vi "探头数据读取.vi"(11 "编号":string) -> ()   [LabVIEW 2016, in "斯坦道多参数.lvlib"]
panel:
  out "日期/时间字符串 2":string
  out "日期/时间字符串":string
  out "运行状态":u16(ring) items=["空闲", "水样测试", "标样核查"]
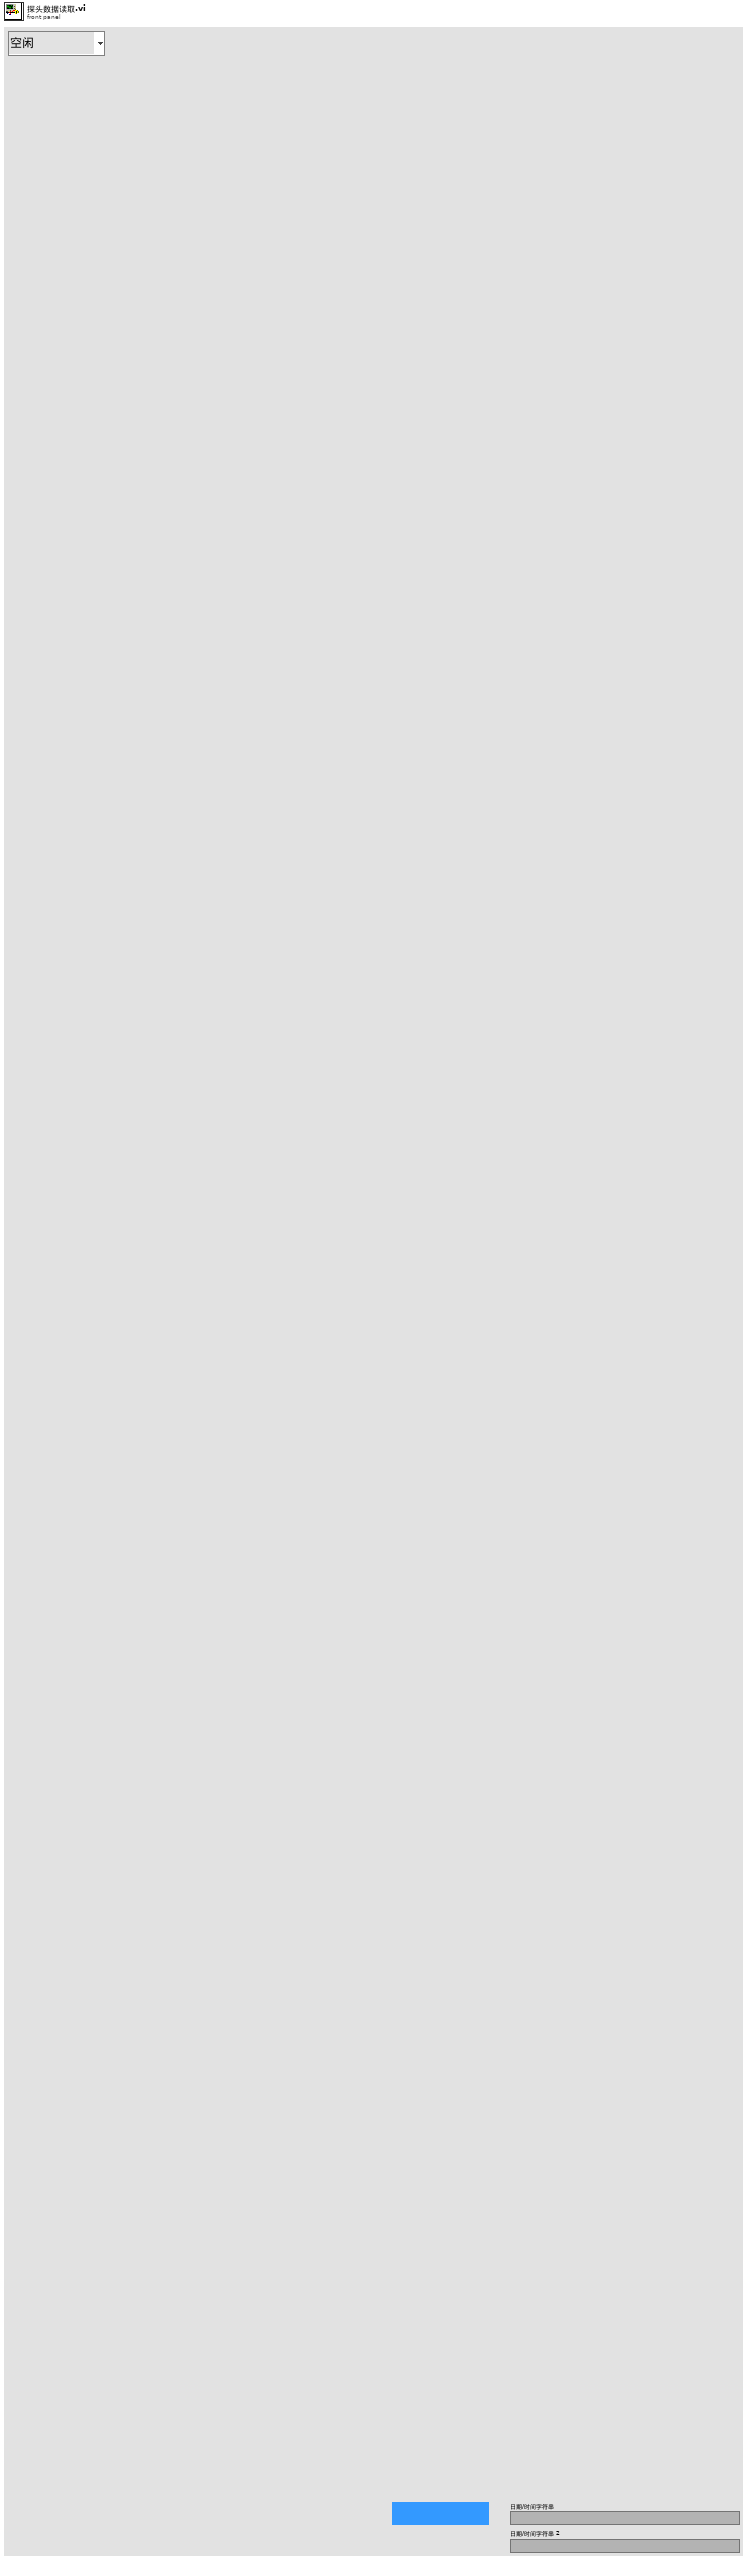
[diagram p1: front panel]
types:
  T1 = typedef "斯坦道多参数.lvlib/通知队列类型.ctl" = enum16{"pH", "DO", "DO2", "Cond", "Turb", "ORP", "叶绿素a", "藻密度", "COD", "氯化物", "氨氮", "水中油"}
  T2 = cluster{"温度测量值":sgl, "测量值":sgl, "温度偏移修正值":sgl, "信号值":sgl, "数据标识":string}
  T3 = cluster{"温度测量值":sgl, "DO%":sgl, "DOmg/L":sgl, "温度偏移修正值":sgl, "数据标识mg/L":string, "数据标识%":string}
  T4 = cluster{"水温 (℃)":cluster{"量程下限":dbl, "量程上限":dbl}, "DO (mg/L)":cluster{"量程下限":dbl, "量程上限":dbl}, "DO (%)":cluster{"量程下限":dbl, "量程上限":dbl}, "pH":cluster{"量程下限":dbl, "量程上限":dbl}, "电导率 (μS/cm)":cluster{"量程下限":dbl, "量程上限":dbl}, "盐度":cluster{"量程下限":dbl, "量程上限":dbl}, "浊度 (NTU)":cluster{"量程下限":dbl, "量程上限":dbl}, "叶绿素a (μg/L)":cluster{"量程下限":dbl, "量程上限":dbl}, "藻密度 (cells/mL)":cluster{"量程下限":dbl, "量程上限":dbl}, "ORP (mV)":cluster{"量程下限":dbl, "量程上限":dbl}, "氯化物（mg/L）":cluster{"量程下限":dbl, "量程上限":dbl}, "COD":cluster{"量程下限":dbl, "量程上限":dbl}, "氨氮":cluster{"量程下限":dbl, "量程上限":dbl}, "水中油":cluster{"量程下限":dbl, "量程上限":dbl}}
  T5 = cluster{"CH":u16, "监测值":dbl, "信号值":sgl, "数据标识":string}
  T6 = typedef "斯坦道多参数.lvlib/探头类型.ctl" = enum16{"禹山", "国弘", "纳清", "STD"}
  T7 = cluster{"pH探头选择":T6, "DO探头选择":T6, "电导率探头选择":T6, "浊度探头选择":T6, "叶绿素a探头选择":T6, "蓝绿藻探头选择":T6, "orp探头选择":T6, "COD探头选择":T6, "DO2探头选择":T6, "氨氮探头选择":T6, "水中油探头选择":T6}
  T8 = cluster{"电极状态标志":u16, "电极型号标志":u16, "酸碱度测量值":sgl, "温度测量值":sgl, "酸碱度信号值":sgl, "温度信号值":sgl, "酸碱度偏移修正值":sgl, "温度偏移修正值":sgl, "手动温度补偿值":sgl, "酸碱度电极零点":sgl, "酸碱度电极斜率":sgl, "第1点标准值记录":sgl, "第1点信号值记录":sgl, "第1点温度值记录":sgl, "第2点标准值记录":sgl, "第2点信号值记录":sgl, "第2点温度值记录":sgl, "命令滤波设定":u16, "温度模式":enum16{"ATC", "MTC"}, "生产批次":u16, "电极序号":u16, "串口地址":u16, "串口波特率":enum16{"9600", "19200", "115200"}, "串口校验位":enum16{"NONE", "ODD", "EVEN"}, "串口停止位":enum16{"1bit", "2bit"}, "第一点标准值":sgl, "第二点标准值":sgl}
  T9 = cluster{"报警码":u16, "pH数值":sgl, "0X0003_NC":sgl, "温度数据":sgl, "pH原始信号 mv":sgl, "0X0009_NC":string, "产品名称":string, "序列号":string, "硬件版本":string, "软件版本":string, "通讯地址":u16, "波特率":u16, "设备类型":u16, "0X0026_NC":string, "第一点原始数据":sgl, "第一点校准数据":sgl, "第二点原始数据":sgl, "第二点校准数据":sgl, "探头校准命令":u16, "温度校准参数":sgl, "温度校准命令":u16}
  T10 = cluster{"电极状态标志":u16, "电极型号标志":u16, "电导率测量值":sgl, "温度测量值":sgl, "电导率信号值":sgl, "温度信号值":sgl, "温度补偿系数":sgl, "电导率偏移修正值":sgl, "温度偏移修正值":sgl, "手动温度补偿值":sgl, "电导率电极零点":sgl, "电导率电极斜率":sgl, "命令滤波设定":u16, "温度模式":enum16{"ATC", "MTC"}, "生产批次":u16, "电极序号":u16, "串口地址":u16, "串口波特率":enum16{"9600", "19200", "115200"}, "串口校验位":enum16{"NONE", "ODD", "EVEN"}, "串口停止位":enum16{"1bit", "2bit"}, "第一点标准值":sgl, "第二点标准值":sgl}
  T11 = cluster{"报警码":u16, "电导率数据（uS/cm）":sgl, "0x0003 NC":sgl, "温度数据":sgl, "电导率原始信号电阻":sgl, "当前量程":u16, "温度补偿系数":sgl, "0X0009_NC":string, "产品名称":string, "序列号":string, "硬件版本":string, "软件版本":string, "通讯地址":u16, "波特率":u16, "设备类型":u16, "0X0026_NC":string, "第一点原始数据":sgl, "第一点校准数据":sgl, "0X0035_NC":sgl, "0X0037_NC":sgl, "探头校准命令":u16, "温度校准参数":sgl, "温度校准命令":u16}
  T12 = cluster{"电极状态标志":u16, "电极型号标志":u16, "溶解氧测量值":sgl, "温度测量值":sgl, "溶解氧饱和度值":sgl, "盐度补偿值":sgl, "大气压补偿值":sgl, "溶解氧偏移修正值":sgl, "温度偏移修正值":sgl, "手动温度补偿值":sgl, "溶解氧电极零点":sgl, "溶解氧电极斜率":sgl, "第1点标准值记录":sgl, "第1点信号值记录":sgl, "第1点温度值记录":sgl, "第2点标准值记录":sgl, "第2点信号值记录":sgl, "第2点温度值记录":sgl, "命令滤波设定":u16, "温度模式":enum16{"ATC", "MTC"}, "生产批次":u16, "电极序号":u16, "串口地址":u16, "串口波特率":enum16{"9600", "19200", "115200"}, "串口校验位":enum16{"NONE", "ODD", "EVEN"}, "串口停止位":enum16{"1bit", "2bit"}, "第一点标准值":sgl, "第二点标准值":sgl}
  T13 = cluster{"报警码":u16, "溶解氧数值（mg/L）":sgl, "溶解氧数据（%）":sgl, "温度数据":sgl, "溶解氧原始信号 nA":sgl, "大气压力":sgl, "盐度":sgl, "0X0009_NC":string, "产品名称":string, "序列号":string, "硬件版本":string, "软件版本":string, "通讯地址":u16, "波特率":u16, "设备类型":u16, "0X0026_NC":string, "第一点原始数据":sgl, "0X0033 NC":sgl, "第二点原始数据":sgl, "0X0037 NC":sgl, "探头校准命令":u16, "温度校准参数":sgl, "温度校准命令":u16}
  T14 = cluster{"电极状态标志":u16, "电极型号标志":u16, "浊度测量值":sgl, "温度测量值":sgl, "浊度信号值":sgl, "浊度偏移修正值":sgl, "温度偏移修正值":sgl, "手动温度补偿值":sgl, "浊度电极零点":sgl, "浊度电极斜率":sgl, "清洁周期":u16, "命令滤波设定":u16, "温度模式":enum16{"ATC", "MTC"}, "生产批次":u16, "电极序号":u16, "串口地址":u16, "串口波特率":enum16{"9600", "19200", "115200"}, "串口校验位":enum16{"NONE", "ODD", "EVEN"}, "串口停止位":enum16{"1bit", "2bit"}, "第一点标准值":sgl, "第二点标准值":sgl, "第三点标准值":sgl}
  T15 = cluster{"报警码":u16, "浊度数值 NTU":sgl, "温度数据":sgl, "原始光强数值":u16, "量程":u16, "平均次数":u16, "清扫模式":u16, "清扫次数":u16, "清扫间隔分钟":u16, "0X000B_NC":string, "产品名称":string, "序列号":string, "硬件版本":string, "软件版本":string, "通讯地址":u16, "波特率":u16, "设备类型":u16, "0X0026_NC":string, "校准量程":u16, "第一点原始光强":u16, "第一点校准数据":sgl, "第二点原始光强":u16, "第二点校准数据":sgl, "第三点原始光强":u16, "第三点校准数据":sgl, "探头校准命令":u16, "温度校准参数":sgl, "温度校准命令":u16}
  T16 = cluster{"电极状态标志":u16, "电极型号标志":u16, "测量值":sgl, "温度测量值":sgl, "信号值":sgl, "温度信号值":sgl, "000AH_NC":sgl, "偏移修正值":sgl, "温度偏移修正值":sgl, "手动温度补偿值":sgl, "命令滤波设定":u16, "温度模式":enum16{"ATC", "MTC"}, "生产批次":u16, "传感器序号":u16, "串口地址":u16, "串口波特率":enum16{"9600", "19200", "115200"}, "串口校验位":enum16{"NONE", "ODD", "EVEN"}, "串口停止位":enum16{"1bit", "2bit"}}
  T17 = cluster{"报警码":u16, "叶绿素a":sgl, "温度数据":sgl, "原始光强数值":u16, "量程":u16, "平均次数":u16, "清扫模式":u16, "清扫次数":u16, "清扫间隔分钟":u16, "0X000B_NC":string, "产品名称":string, "序列号":string, "硬件版本":string, "软件版本":string, "通讯地址":u16, "波特率":u16, "设备类型":u16, "0X0026_NC":string, "校准量程":u16, "第一点原始光强":u16, "第一点校准数据":sgl, "第二点原始光强":u16, "第二点校准数据":sgl, "第三点原始光强":u16, "第三点校准数据":sgl, "探头校准命令":u16, "温度校准参数":sgl, "温度校准命令":u16}
  T18 = cluster{"报警码":u16, "蓝绿藻":sgl, "温度数据":sgl, "原始光强数值":u16, "0X0006_NC":u16, "平均次数":u16, "清扫模式":u16, "清扫次数":u16, "清扫间隔分钟":u16, "0X000B_NC":string, "产品名称":string, "序列号":string, "硬件版本":string, "软件版本":string, "通讯地址":u16, "波特率":u16, "设备类型":u16, "0X0026_NC":string, "0X0030_NC":u16, "第一点原始光强":u16, "第一点校准数据":sgl, "第二点原始光强":u16, "第二点校准数据":sgl, "第三点原始光强":u16, "第三点校准数据":sgl, "探头校准命令":u16, "温度校准参数":sgl, "温度校准命令":u16}
  T19 = cluster{"电极状态标志":u16, "电极型号标志":u16, "COD测量值":sgl, "浊度测量值":sgl, "COD信号值":sgl, "浊度信号值":sgl, "温度测量值":sgl, "COD偏移修正值":sgl, "浊度偏移修正值":sgl, "COD水样校正值":sgl, "温度偏移修正值":sgl, "COD零点系数":sgl, "COD斜率系数":sgl, "浊度零点系数":sgl, "浊度斜率系数":sgl, "COD测值K值":sgl, "浊度测值K值":sgl, "浊度补偿COD系数值":sgl, "COD温度补偿系数值 ":sgl, "测量周期":u16, "清洗周期":u16, "命令寄存器":u16, "数字滤波设定":u16, "温度模式":enum16{"AUTO", "OFF"}, "生产批次":u16, "电极序号":u16, "串口地址":u16, "串口波特率":enum16{"9600", "19200", "115200"}, "串口校验位":enum16{"NONE", "ODD", "EVEN"}, "串口停止位":enum16{"1bit", "2bit"}, "第一点校正指令":u16, "第一点标准值":sgl, "第二点校正指令":u16, "第二点标准值":sgl, "第三点校正指令":u16, "第三点标准值":sgl, "COD吸光度":sgl, "浊度吸光度":sgl, "温度信号值":sgl}
  T20 = cluster{"电极状态标志":u16, "电极型号标志":u16, "测量值":sgl, "温度测量值":sgl, "信号值":sgl, "温度信号值":sgl, "偏移修正值":sgl, "温度偏移修正值":sgl, "手动温度补偿值":sgl, "电极零点":sgl, "电极斜率":sgl, "第1点标准值记录":sgl, "第1点信号值记录":sgl, "第1点温度值记录":sgl, "第2点标准值记录":sgl, "第2点信号值记录":sgl, "第2点温度值记录":sgl, "命令滤波设定":u16, "温度模式":enum16{"ATC", "MTC"}, "生产批次":u16, "电极序号":u16, "串口地址":u16, "串口波特率":enum16{"9600", "19200", "115200"}, "串口校验位":enum16{"NONE", "ODD", "EVEN"}, "串口停止位":enum16{"1bit", "2bit"}, "第一点标准值":sgl, "第二点标准值":sgl}
  T21 = cluster{"电极状态标志":u16, "电极型号标志":u16, "测量值":sgl, "温度测量值":sgl, "信号值":sgl, "水中油B值":sgl, "温度B值":sgl, "水中油零点系数":sgl, "水中油斜率系数":sgl, "水中油K值":sgl, "空白电位值":sgl, "温度信号值":sgl, "温度补偿系数":sgl, "测量档位":u16, "清洁周期":u16, "命令寄存器":u16, "数位滤波设定":u16, "温度模式":enum16{"ATC", "MTC"}, "生产批次":u16, "电极序号":u16, "串口地址":u16, "串口波特率":enum16{"9600", "19200", "115200"}, "串口校验位":enum16{"NONE", "ODD", "EVEN"}, "串口停止位":enum16{"1bit", "2bit"}, "第一点校正指令":u16, "第一点标准值":sgl, "第二点校正指令":u16, "第二点标准值":sgl, "第三点校正指令":u16, "第三点标准值":sgl}
  T22 = cluster{"报警码":u16, "参数1数据":sgl, "参数2数据":sgl, "参数3数据":sgl, "参数4数据":sgl, "温度数据":sgl, "参数1原始信号":sgl, "参数2原始信号":sgl, "参数3原始信号":sgl, "参数4原始信号":sgl, "序列号":string, "硬件版本":string, "软件版本":string, "通讯地址":u16, "波特率":u16, "设备类型":u16, "0X0026_NC":string, "校准参数类型":u16, "第一点原始数据":sgl, "第一点校准数据":sgl, "第二点原始数据":sgl, "第二点校准数据":sgl, "探头校准命令":u16, "温度校准参数":sgl, "温度校准命令":u16}
  T23 = cluster{"ph":bool, "DO":bool, "Cond":bool, "Turb":bool, "叶绿素a":bool, "藻密度":bool, "ORP":bool, "cod":bool, "DO2":bool, "氯化物":bool, "氨氮":bool, "水中油":bool}
  T24 = cluster{"ph":bool, "DO":bool, "Cond":bool, "Turb":bool, "叶绿素a":bool, "藻密度":bool, "ORP":bool, "COD":bool, "DO2":bool, "氯化物":bool, "氨氮":bool, "水中油":bool}
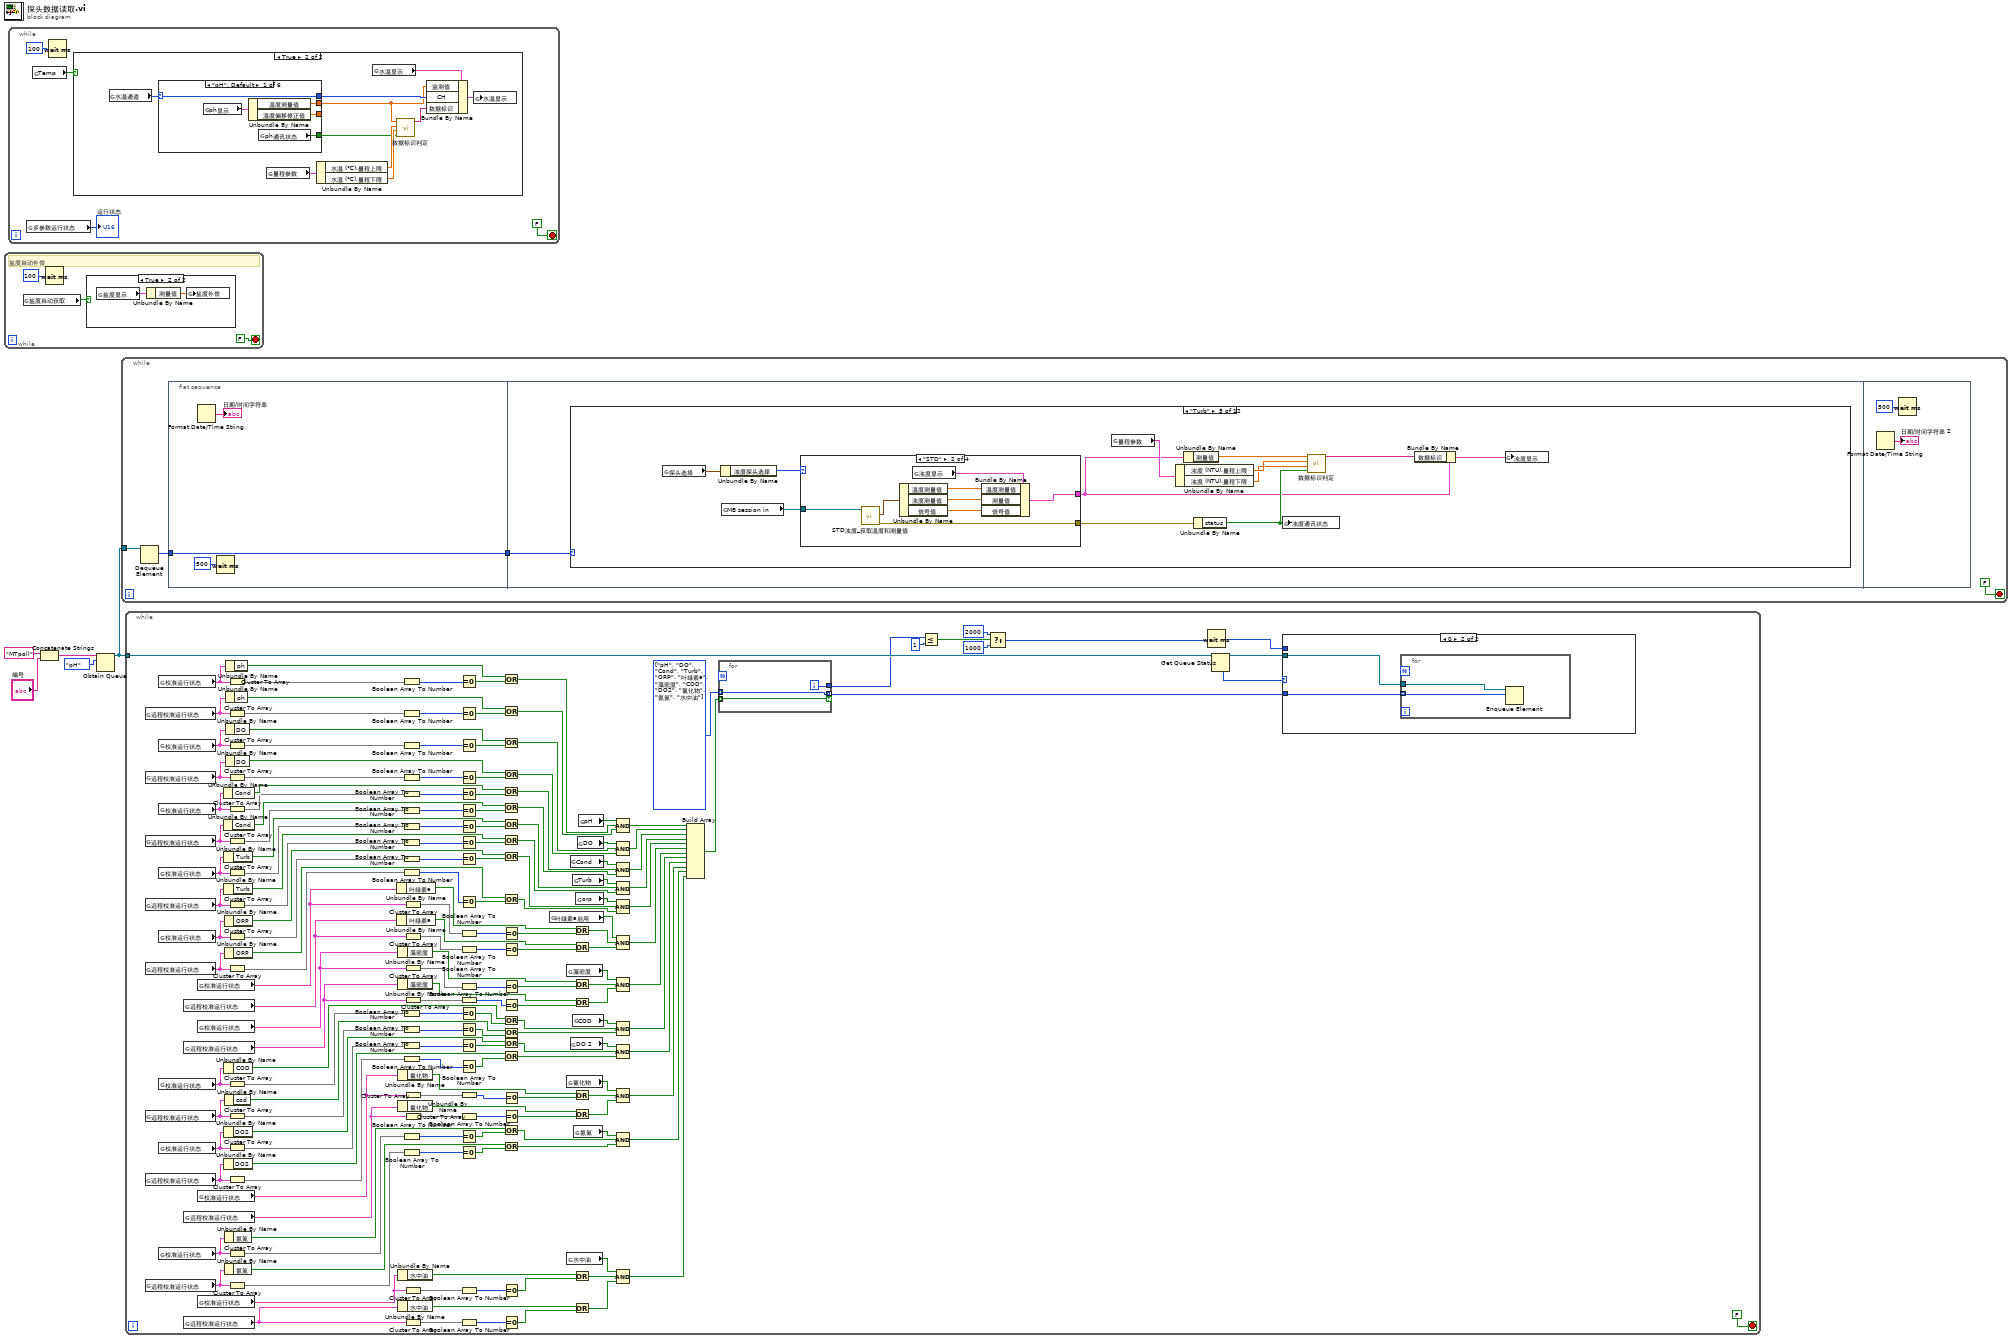
[diagram p0: block diagram]
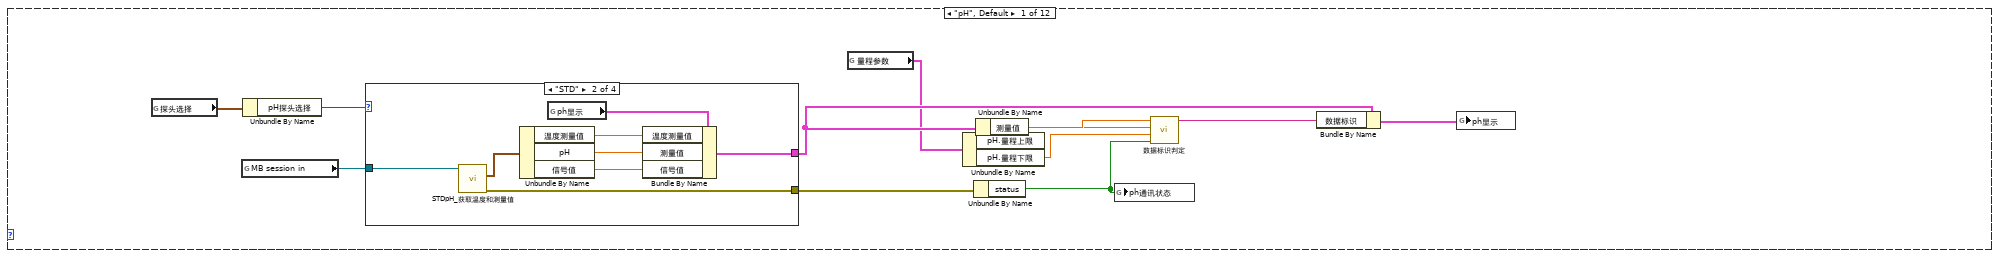
[diagram p3: hidden frame]
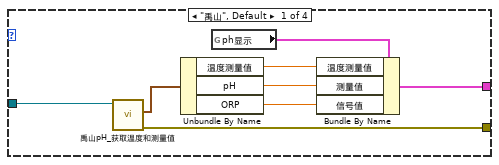
[diagram p4: hidden frame]
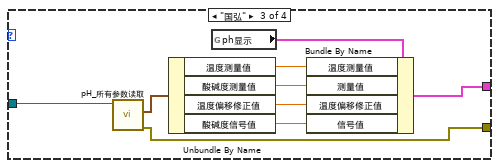
[diagram p5: hidden frame]
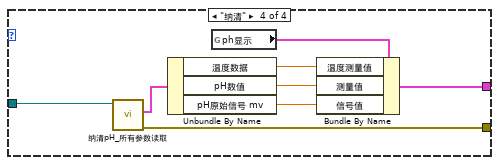
[diagram p6: hidden frame]
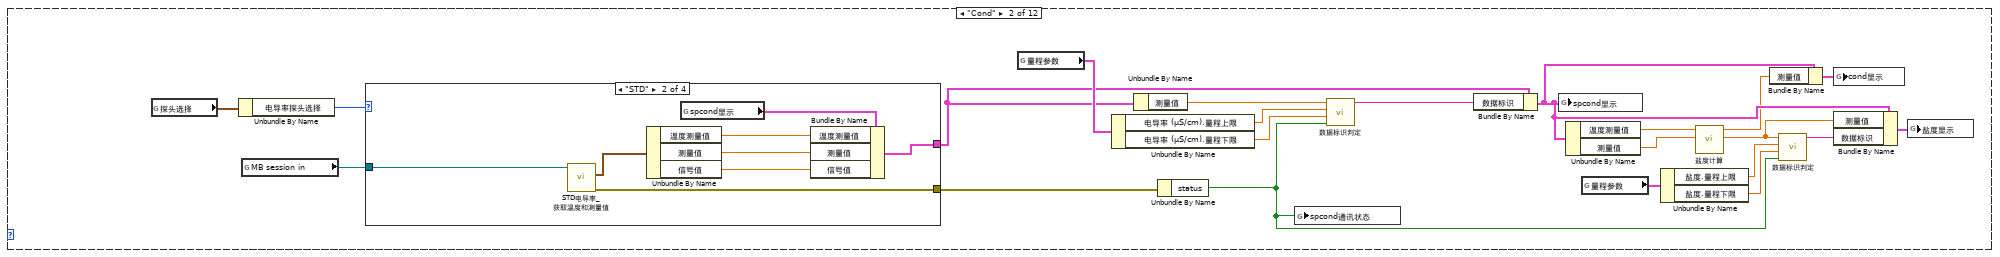
[diagram p7: hidden frame]
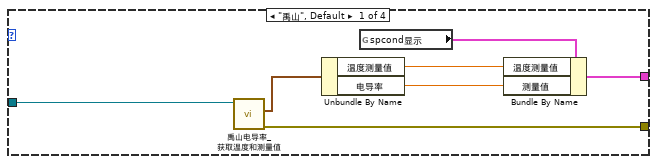
[diagram p8: hidden frame]
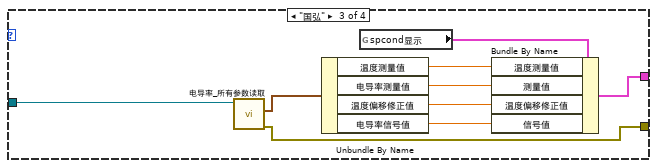
[diagram p9: hidden frame]
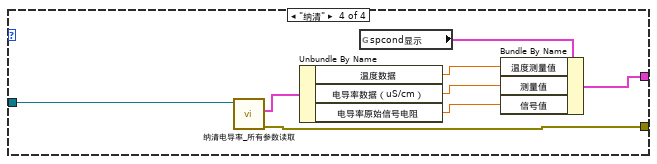
[diagram p10: hidden frame]
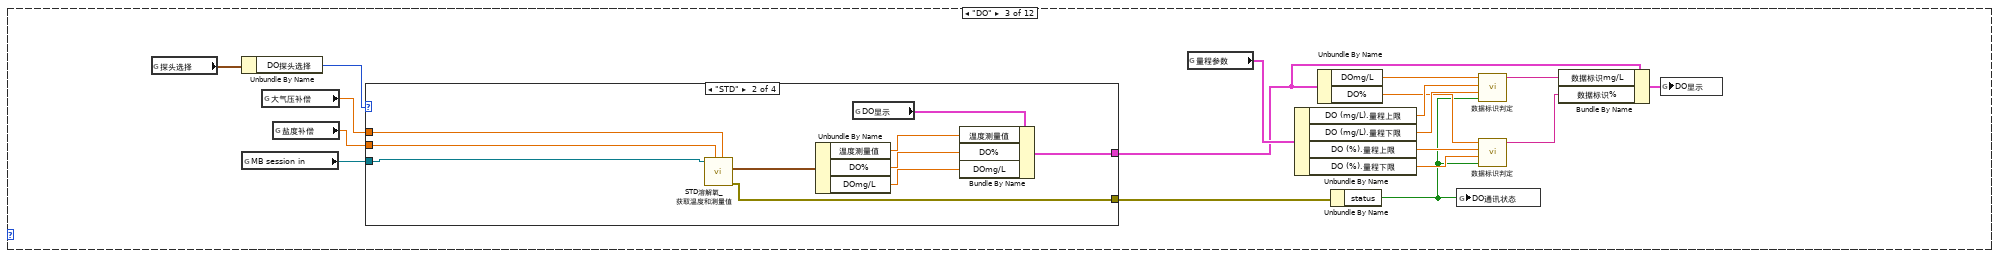
[diagram p11: hidden frame]
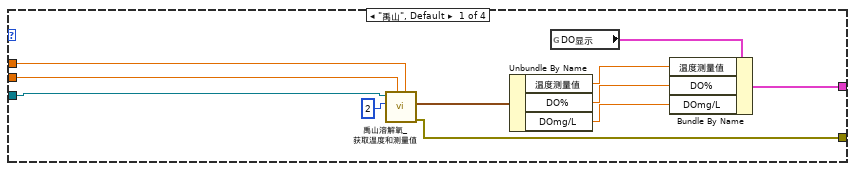
[diagram p12: hidden frame]
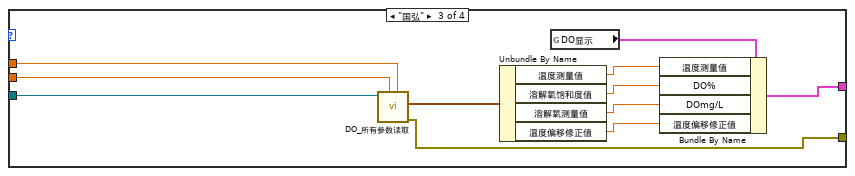
[diagram p13: hidden frame]
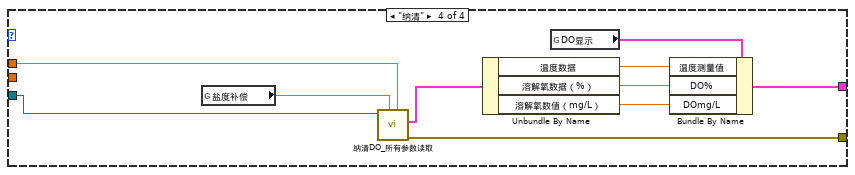
[diagram p14: hidden frame]
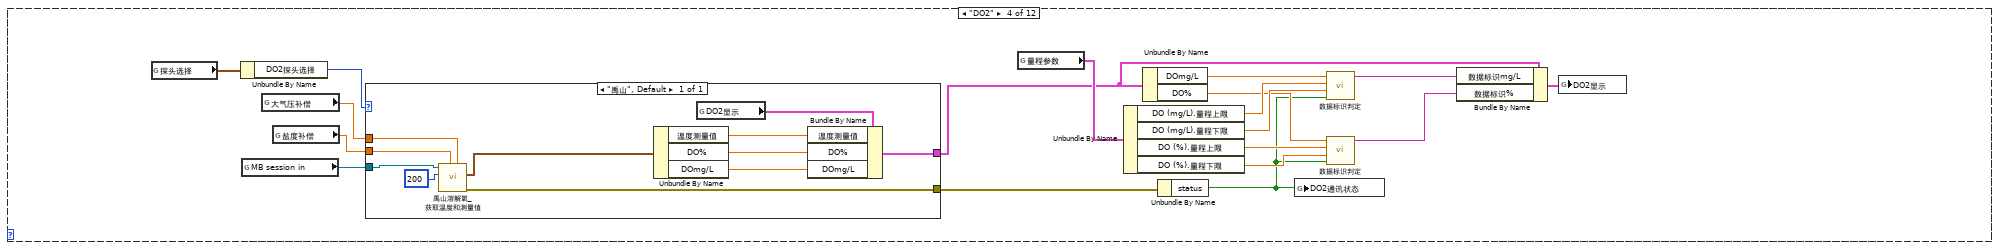
[diagram p15: hidden frame]
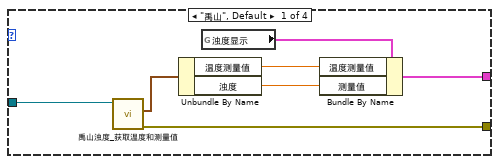
[diagram p16: hidden frame]
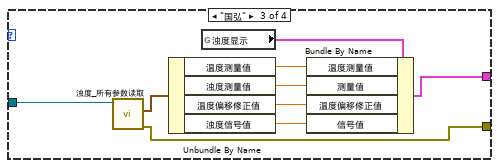
[diagram p17: hidden frame]
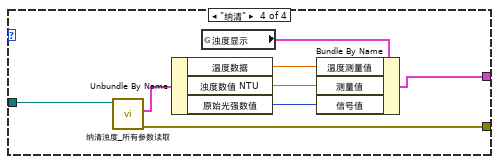
[diagram p18: hidden frame]
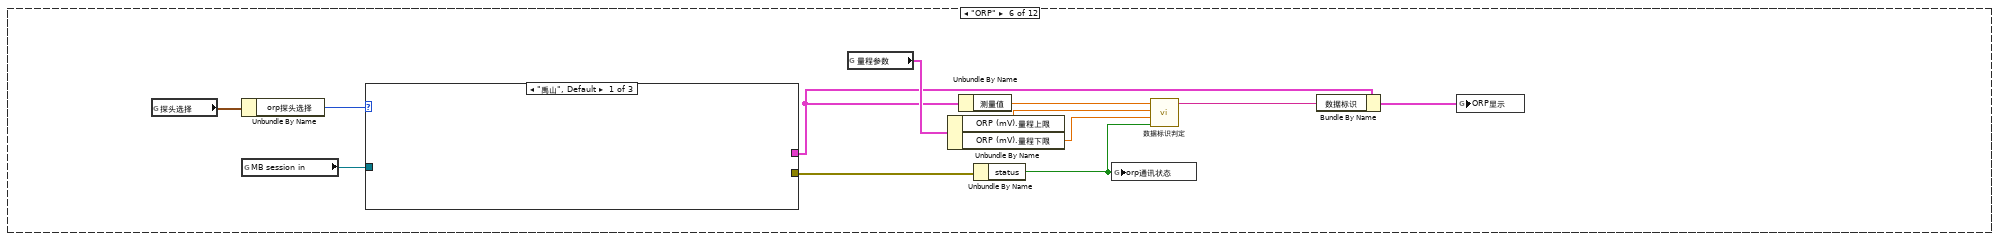
[diagram p19: hidden frame]
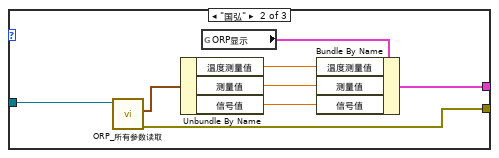
[diagram p20: hidden frame]
diagram:
  n1 = while {
    stop <- FALSE stop-if-true
    # "盐度自动补偿"
    n2 = global read "断电保存变量.vi" "盐度自动获取"() -> (w7:bool)
    n3 = Wait (ms)(milliseconds to wait=u32 100 ("等待时间（毫秒）")) -> ()  [unwired: 1 out]
    n4 = case shown="True" w7 {
      frame False {
      }
      frame True {
        n5 = global read "多参数全局变量.vi" "盐度显示"() -> (w10:T2)
        n6 = Unbundle By Name(w10) -> ("测量值"=w9:sgl)
        n7 = global write "断电保存变量.vi" "盐度补偿"(w9) -> ()
      }
    }
  }
  n8 = while {
    stop <- FALSE stop-if-true
    n9 = global read "多参数全局变量.vi" "多参数运行状态"() -> (→"运行状态":u16)
    n10 = global read "断电保存变量.vi" "Temp"() -> (w12:bool)
    n11 = Wait (ms)(milliseconds to wait=u32 100 ("等待时间（毫秒）")) -> ()  [unwired: 1 out]
    n12 = case shown="True" w12 {
      frame False {
      }
      frame True {
        n13 = global read "断电保存变量.vi" "水温通道"() -> (w24:enum16{"pH", "DO", "浊度", "电导率", "叶绿素a", "藻密度"})
        n14 = case shown="\"pH\", Default" w24 {
          selector: w24 -> [w29 w34 w39 w44 w49 w54]
          tunnel: [w29 w34 w39 w44 w49 w54] -> w23
          tunnel: [w27 w31 w36 w41 w46 w51] -> _
          tunnel: [w28 w32 w37 w42 w47 w52] -> w17
          tunnel: [w25 w30 w35 w40 w45 w50] -> w15
          frame "pH", Default {
            n15 = global read "多参数全局变量.vi" "ph显示"() -> (w26:T2)
            n16 = Unbundle By Name(w26) -> ("温度测量值"=w28:sgl, "温度偏移修正值"=w27:sgl)
            n17 = global read "多参数全局变量.vi" "ph通讯状态"() -> (w25:bool)
          }
          frame "电导率" {
            n18 = global read "多参数全局变量.vi" "spcond显示"() -> (w33:T2)
            n19 = global read "多参数全局变量.vi" "spcond通讯状态"() -> (w30:bool)
            n20 = Unbundle By Name(w33) -> ("温度测量值"=w32:sgl, "温度偏移修正值"=w31:sgl)
          }
          frame "DO" {
            n21 = global read "多参数全局变量.vi" "DO显示"() -> (w38:T3)
            n22 = Unbundle By Name(w38) -> ("温度测量值"=w37:sgl, "温度偏移修正值"=w36:sgl)
            n23 = global read "多参数全局变量.vi" "DO通讯状态"() -> (w35:bool)
          }
          frame "浊度" {
            n24 = global read "多参数全局变量.vi" "浊度显示"() -> (w43:T2)
            n25 = Unbundle By Name(w43) -> ("温度测量值"=w42:sgl, "温度偏移修正值"=w41:sgl)
            n26 = global read "多参数全局变量.vi" "浊度通讯状态"() -> (w40:bool)
          }
          frame "叶绿素a" {
            n27 = global read "多参数全局变量.vi" "叶绿素a显示"() -> (w48:T2)
            n28 = global read "多参数全局变量.vi" "叶绿素a通讯状态"() -> (w45:bool)
            n29 = Unbundle By Name(w48) -> ("温度测量值"=w47:sgl, "温度偏移修正值"=w46:sgl)
          }
          frame "藻密度" {
            n30 = global read "多参数全局变量.vi" "藻密度显示"() -> (w53:T2)
            n31 = global read "多参数全局变量.vi" "藻密度通讯状态"() -> (w50:bool)
            n32 = Unbundle By Name(w53) -> ("温度测量值"=w52:sgl, "温度偏移修正值"=w51:sgl)
          }
        }
        n33 = global read "断电保存变量.vi" "量程参数"() -> (w20:T4)
        n34 = Unbundle By Name(w20) -> ("水温 (℃).量程上限"=w18:dbl, "水温 (℃).量程下限"=w19:dbl)
        n35 = global read "多参数全局变量.vi" "水温显示"() -> (w21:T5)
        n36 = call "数据标识判定.vi"("通讯故障"=w15, "量程下限"=w19, "量程上限"=w18, "测量值"=w17) -> ("数据标识"=w16:string)  [unwired: 7 in]
        n37 = Bundle By Name(cluster=w21, "监测值"=w17, "CH"=w23, "数据标识"=w16) -> (w22:T5)
        n38 = global write "多参数全局变量.vi" "水温显示"(w22) -> ()
      }
    }
  }
  n39 = Concatenate Strings("MTpoll" ("名称（未命名）"), "编号") -> (w3:string)
  n40 = Obtain Queue(name (unnamed)=w3, element data type=通知队列类型."pH" ("枚举")) -> (queue out=w1:refnum<queue>)  [unwired: 3 in, 2 out]
  n41 = while {
    tunnel: w1 -> [w58]
    stop <- FALSE stop-if-true
    n42 = Dequeue Element(queue=w58) -> (element=w57:T1)  [unwired: 2 in, 3 out]
    n43 = flat-sequence {
      tunnel: w57 -> [w61]
      tunnel: [w61] -> w55
      tunnel: w55 -> [w62]
      frame #0 {
        n44 = Format Date/Time String() -> (date/time string=→"日期/时间字符串":string)  [unwired: 3 in]
        n45 = Wait (ms)(milliseconds to wait=u32 500 ("等待时间（毫秒）")) -> ()  [unwired: 1 out]
      }
      frame #1 {
        n46 = case shown="\"Turb\"" w62 {
          frame "pH", Default {
            n47 = global read "断电保存变量.vi" "探头选择"() -> (w74:T7)
            n48 = global read "多参数全局变量.vi" "MB session in"() -> (w72:refnum<class "MB_Master.lvclass">)
            n49 = Unbundle By Name(w74) -> ("pH探头选择"=w73:T6)
            n50 = case shown="\"STD\"" w73 {
              tunnel: w72 -> [w82 w90 w99 w105]
              tunnel: [w81 w89 w98 w103] -> w71
              tunnel: [w79 w87 w95 w106] -> w70
              frame "禹山", Default {
                n51 = call "禹山pH_获取温度和测量值.vi"("MB session in"=w82) -> ("error out"=w81:errorcluster, "输出值"=w78:cluster{"温度测量值":sgl, "ORP":sgl, "pH":sgl})  [unwired: 8 in, 1 out]
                n52 = Unbundle By Name(w78) -> ("温度测量值"=w77:sgl, "pH"=w76:sgl, "ORP"=w75:sgl)
                n53 = global read "多参数全局变量.vi" "ph显示"() -> (w80:T2)
                n54 = Bundle By Name(cluster=w80, "温度测量值"=w77, "测量值"=w76, "信号值"=w75) -> (w79:T2)
              }
              frame "STD" {
                n55 = call "STDpH_获取温度和测量值.vi"("MB session in"=w90) -> ("error out"=w89:errorcluster, "STDpH"=w83:cluster{"温度测量值":sgl, "pH":sgl, "信号值":sgl})  [unwired: 8 in, 1 out]
                n56 = Unbundle By Name(w83) -> ("温度测量值"=w86:sgl, "pH"=w85:sgl, "信号值"=w84:sgl)
                n57 = global read "多参数全局变量.vi" "ph显示"() -> (w88:T2)
                n58 = Bundle By Name(cluster=w88, "温度测量值"=w86, "测量值"=w85, "信号值"=w84) -> (w87:T2)
              }
              frame "国弘" {
                n59 = call "pH_所有参数读取.vi"("MB session in"=w99) -> ("error out"=w98:errorcluster, "输出值"=w97:T8)  [unwired: 8 in, 1 out]
                n60 = Unbundle By Name(w97) -> ("温度测量值"=w92:sgl, "酸碱度测量值"=w93:sgl, "温度偏移修正值"=w94:sgl, "酸碱度信号值"=w91:sgl)
                n61 = global read "多参数全局变量.vi" "ph显示"() -> (w96:T2)
                n62 = Bundle By Name(cluster=w96, "温度测量值"=w92, "测量值"=w93, "温度偏移修正值"=w94, "信号值"=w91) -> (w95:T2)
              }
              frame "纳清" {
                n63 = call "纳清pH_所有参数读取.vi"("MB session in"=w105) -> ("error out"=w103:errorcluster, "输出值"=w104:T9)  [unwired: 8 in, 1 out]
                n64 = Unbundle By Name(w104) -> ("温度数据"=w102:sgl, "pH数值"=w101:sgl, "pH原始信号 mv"=w100:sgl)
                n65 = global read "多参数全局变量.vi" "ph显示"() -> (w107:T2)
                n66 = Bundle By Name(cluster=w107, "温度测量值"=w102, "测量值"=w101, "信号值"=w100) -> (w106:T2)
              }
            }
            n67 = global read "断电保存变量.vi" "量程参数"() -> (w69:T4)
            n68 = Unbundle By Name(w69) -> ("pH.量程上限"=w67:dbl, "pH.量程下限"=w66:dbl)
            n69 = Unbundle By Name(w71) -> ("status"=w65:bool)
            n70 = Unbundle By Name(w70) -> ("测量值"=w68:sgl)
            n71 = global write "多参数全局变量.vi" "ph通讯状态"(w65) -> ()
            n72 = call "数据标识判定.vi"("通讯故障"=w65, "量程下限"=w66, "量程上限"=w67, "测量值"=w68) -> ("数据标识"=w63:string)  [unwired: 7 in]
            n73 = Bundle By Name(cluster=w70, "数据标识"=w63) -> (w64:T2)
            n74 = global write "多参数全局变量.vi" "ph显示"(w64) -> ()
          }
          frame "Cond" {
            n75 = global read "断电保存变量.vi" "探头选择"() -> (w129:T7)
            n76 = Unbundle By Name(w129) -> ("电导率探头选择"=w128:T6)
            n77 = global read "多参数全局变量.vi" "MB session in"() -> (w127:refnum<class "MB_Master.lvclass">)
            n78 = case shown="\"STD\"" w128 {
              tunnel: w127 -> [w136 w144 w153 w157]
              tunnel: [w130 w138 w151 w160] -> w122
              tunnel: [w135 w143 w150 w155] -> w126
              frame "禹山", Default {
                n79 = call "禹山电导率_获取温度和测量值.vi"("MB session in"=w136) -> ("error out"=w135:errorcluster, "输出值"=w133:cluster{"温度测量值":sgl, "电导率":sgl, "错误标志":u16})  [unwired: 8 in, 1 out]
                n80 = Unbundle By Name(w133) -> ("温度测量值"=w132:sgl, "电导率"=w131:sgl)
                n81 = global read "多参数全局变量.vi" "spcond显示"() -> (w134:T2)
                n82 = Bundle By Name(cluster=w134, "温度测量值"=w132, "测量值"=w131) -> (w130:T2)
              }
              frame "STD" {
                n83 = call "STD电导率_获取温度和测量值.vi"("MB session in"=w144) -> ("error out"=w143:errorcluster, "STDspcond"=w141:cluster{"温度测量值":sgl, "测量值":sgl, "信号值":sgl})  [unwired: 8 in, 1 out]
                n84 = Unbundle By Name(w141) -> ("温度测量值"=w140:sgl, "测量值"=w139:sgl, "信号值"=w137:sgl)
                n85 = global read "多参数全局变量.vi" "spcond显示"() -> (w142:T2)
                n86 = Bundle By Name(cluster=w142, "温度测量值"=w140, "测量值"=w139, "信号值"=w137) -> (w138:T2)
              }
              frame "国弘" {
                n87 = call "电导率_所有参数读取.vi"("MB session in"=w153) -> ("error out"=w150:errorcluster, "输出值"=w149:T10)  [unwired: 8 in, 1 out]
                n88 = Unbundle By Name(w149) -> ("温度测量值"=w148:sgl, "电导率测量值"=w147:sgl, "温度偏移修正值"=w146:sgl, "电导率信号值"=w145:sgl)
                n89 = global read "多参数全局变量.vi" "spcond显示"() -> (w152:T2)
                n90 = Bundle By Name(cluster=w152, "温度测量值"=w148, "测量值"=w147, "温度偏移修正值"=w146, "信号值"=w145) -> (w151:T2)
              }
              frame "纳清" {
                n91 = call "纳清电导率_所有参数读取.vi"("MB session in"=w157) -> ("error out"=w155:errorcluster, "输出值"=w156:T11)  [unwired: 8 in, 1 out]
                n92 = Unbundle By Name(w156) -> ("温度数据"=w159:sgl, "电导率数据（uS/cm）"=w158:sgl, "电导率原始信号电阻"=w154:sgl)
                n93 = global read "多参数全局变量.vi" "spcond显示"() -> (w161:T2)
                n94 = Bundle By Name(cluster=w161, "温度测量值"=w159, "测量值"=w158, "信号值"=w154) -> (w160:T2)
              }
            }
            n95 = global read "断电保存变量.vi" "量程参数"() -> (w125:T4)
            n96 = Unbundle By Name(w125) -> ("电导率 (μS/cm).量程上限"=w124:dbl, "电导率 (μS/cm).量程下限"=w123:dbl)
            n97 = Unbundle By Name(w122) -> ("测量值"=w121:sgl)
            n98 = Unbundle By Name(w126) -> ("status"=w118:bool)
            n99 = global write "多参数全局变量.vi" "spcond通讯状态"(w118) -> ()
            n100 = call "数据标识判定.vi"("通讯故障"=w118, "量程下限"=w123, "量程上限"=w124, "测量值"=w121) -> ("数据标识"=w119:string)  [unwired: 7 in]
            n101 = Bundle By Name(cluster=w122, "数据标识"=w119) -> (w120:T2)
            n102 = global write "多参数全局变量.vi" "spcond显示"(w120) -> ()
            n103 = Unbundle By Name(w120) -> ("温度测量值"=w117:sgl, "测量值"=w116:sgl)
            n104 = global read "断电保存变量.vi" "量程参数"() -> (w110:T4)
            n105 = Unbundle By Name(w110) -> ("盐度.量程上限"=w111:dbl, "盐度.量程下限"=w112:dbl)
            n106 = call "盐度计算.vi"("spCond"=w116, "Temp"=w117) -> ("saltresult"=w109:dbl, "cond"=w115:dbl)  [unwired: 8 in]
            n107 = Bundle By Name(cluster=w120, "测量值"=w115) -> (w114:T2)
            n108 = call "数据标识判定.vi"("通讯故障"=w118, "量程下限"=w112, "量程上限"=w111, "测量值"=w109) -> ("数据标识"=w108:string)  [unwired: 7 in]
            n109 = global write "多参数全局变量.vi" "cond显示"(w114) -> ()
            n110 = Bundle By Name(cluster=w120, "测量值"=w109, "数据标识"=w108) -> (w113:T2)
            n111 = global write "多参数全局变量.vi" "盐度显示"(w113) -> ()
          }
          frame "DO" {
            n112 = global read "断电保存变量.vi" "探头选择"() -> (w179:T7)
            n113 = Unbundle By Name(w179) -> ("DO探头选择"=w178:T6)
            n114 = global read "多参数全局变量.vi" "MB session in"() -> (w177:refnum<class "MB_Master.lvclass">)
            n115 = global read "断电保存变量.vi" "大气压补偿"() -> (w162:dbl)
            n116 = global read "断电保存变量.vi" "盐度补偿"() -> (w163:dbl)
            n117 = case shown="\"STD\"" w178 {
              tunnel: w177 -> [w190 w200 w211 w216]
              tunnel: [w188 w198 w209 w220] -> w170
              tunnel: [w180 w191 w204 w214] -> w176
              tunnel: w163 -> [w182 w193 w202 _]
              tunnel: w162 -> [w181 w192 w201 w212]
              frame "禹山", Default {
                n118 = call "禹山溶解氧_获取温度和测量值.vi"("大气压补偿"=w181, "盐度补偿"=w182, "salve ID"=u16 2, "MB session in"=w190) -> ("error out"=w180:errorcluster, "输出值"=w184:cluster{"温度测量值":sgl, "DO%":sgl, "DOmg/L":sgl})  [unwired: 5 in, 1 out]
                n119 = Unbundle By Name(w184) -> ("温度测量值"=w187:sgl, "DO%"=w186:sgl, "DOmg/L"=w185:sgl)
                n120 = global read "多参数全局变量.vi" "DO显示"() -> (w189:T3)
                n121 = Bundle By Name(cluster=w189, "温度测量值"=w187, "DO%"=w186, "DOmg/L"=w185) -> (w188:T3)
              }
              frame "STD" {
                n122 = call "STD溶解氧_获取温度和测量值.vi"("大气压补偿"=w192, "盐度补偿"=w193, "MB session in"=w200) -> ("error out"=w191:errorcluster, "输出值"=w194:cluster{"温度测量值":sgl, "DO%":sgl, "DOmg/L":sgl})  [unwired: 6 in, 1 out]
                n123 = Unbundle By Name(w194) -> ("温度测量值"=w197:sgl, "DO%"=w196:sgl, "DOmg/L"=w195:sgl)
                n124 = global read "多参数全局变量.vi" "DO显示"() -> (w199:T3)
                n125 = Bundle By Name(cluster=w199, "温度测量值"=w197, "DO%"=w196, "DOmg/L"=w195) -> (w198:T3)
              }
              frame "国弘" {
                n126 = call "DO_所有参数读取.vi"("大气压补偿"=w201, "盐度补偿"=w202, "MB session in"=w211) -> ("error out"=w204:errorcluster, "输出值"=w208:T12)  [unwired: 6 in, 1 out]
                n127 = Unbundle By Name(w208) -> ("温度测量值"=w205:sgl, "溶解氧饱和度值"=w206:sgl, "溶解氧测量值"=w207:sgl, "温度偏移修正值"=w203:sgl)
                n128 = global read "多参数全局变量.vi" "DO显示"() -> (w210:T3)
                n129 = Bundle By Name(cluster=w210, "温度测量值"=w205, "DO%"=w206, "DOmg/L"=w207, "温度偏移修正值"=w203) -> (w209:T3)
              }
              frame "纳清" {
                n130 = global read "断电保存变量.vi" "盐度补偿"() -> (w213:dbl)
                n131 = call "纳清DO_所有参数读取.vi"("大气压补偿"=w212, "盐度补偿"=w213, "MB session in"=w216) -> ("error out"=w214:errorcluster, "输出值"=w215:T13)  [unwired: 6 in, 1 out]
                n132 = Unbundle By Name(w215) -> ("温度数据"=w217:sgl, "溶解氧数据（%）"=w218:sgl, "溶解氧数值（mg/L）"=w219:sgl)
                n133 = global read "多参数全局变量.vi" "DO显示"() -> (w221:T3)
                n134 = Bundle By Name(cluster=w221, "温度测量值"=w217, "DO%"=w218, "DOmg/L"=w219) -> (w220:T3)
              }
            }
            n135 = global read "断电保存变量.vi" "量程参数"() -> (w175:T4)
            n136 = Unbundle By Name(w175) -> ("DO (mg/L).量程上限"=w174:dbl, "DO (mg/L).量程下限"=w173:dbl, "DO (%).量程上限"=w172:dbl, "DO (%).量程下限"=w171:dbl)
            n137 = Unbundle By Name(w170) -> ("DOmg/L"=w169:sgl, "DO%"=w168:sgl)
            n138 = Unbundle By Name(w176) -> ("status"=w164:bool)
            n139 = global write "多参数全局变量.vi" "DO通讯状态"(w164) -> ()
            n140 = call "数据标识判定.vi"("通讯故障"=w164, "量程下限"=w173, "量程上限"=w174, "测量值"=w169) -> ("数据标识"=w166:string)  [unwired: 7 in]
            n141 = call "数据标识判定.vi"("通讯故障"=w164, "量程下限"=w171, "量程上限"=w172, "测量值"=w168) -> ("数据标识"=w165:string)  [unwired: 7 in]
            n142 = Bundle By Name(cluster=w170, "数据标识mg/L"=w166, "数据标识%"=w165) -> (w167:T3)
            n143 = global write "多参数全局变量.vi" "DO显示"(w167) -> ()
          }
          frame "DO2" {
            n144 = global read "断电保存变量.vi" "探头选择"() -> (w239:T7)
            n145 = Unbundle By Name(w239) -> ("DO2探头选择"=w238:T6)
            n146 = global read "多参数全局变量.vi" "MB session in"() -> (w237:refnum<class "MB_Master.lvclass">)
            n147 = global read "断电保存变量.vi" "大气压补偿"() -> (w222:dbl)
            n148 = global read "断电保存变量.vi" "盐度补偿"() -> (w223:dbl)
            n149 = case shown="\"禹山\", Default" w238 {
              tunnel: w237 -> [w250]
              tunnel: [w248] -> w230
              tunnel: [w244] -> w236
              tunnel: w223 -> [w241]
              tunnel: w222 -> [w240]
              frame "禹山", Default {
                n150 = call "禹山溶解氧_获取温度和测量值.vi"("大气压补偿"=w240, "盐度补偿"=w241, "salve ID"=u16 200, "MB session in"=w250) -> ("error out"=w244:errorcluster, "输出值"=w243:cluster{"温度测量值":sgl, "DO%":sgl, "DOmg/L":sgl})  [unwired: 5 in, 1 out]
                n151 = Unbundle By Name(w243) -> ("温度测量值"=w247:sgl, "DO%"=w246:sgl, "DOmg/L"=w245:sgl)
                n152 = global read "多参数全局变量.vi" "DO2显示"() -> (w249:T3)
                n153 = Bundle By Name(cluster=w249, "温度测量值"=w247, "DO%"=w246, "DOmg/L"=w245) -> (w248:T3)
              }
            }
            n154 = global read "断电保存变量.vi" "量程参数"() -> (w235:T4)
            n155 = Unbundle By Name(w235) -> ("DO (mg/L).量程上限"=w234:dbl, "DO (mg/L).量程下限"=w233:dbl, "DO (%).量程上限"=w232:dbl, "DO (%).量程下限"=w231:dbl)
            n156 = Unbundle By Name(w230) -> ("DOmg/L"=w229:sgl, "DO%"=w228:sgl)
            n157 = Unbundle By Name(w236) -> ("status"=w224:bool)
            n158 = global write "多参数全局变量.vi" "DO2通讯状态"(w224) -> ()
            n159 = call "数据标识判定.vi"("通讯故障"=w224, "量程下限"=w233, "量程上限"=w234, "测量值"=w229) -> ("数据标识"=w226:string)  [unwired: 7 in]
            n160 = call "数据标识判定.vi"("通讯故障"=w224, "量程下限"=w231, "量程上限"=w232, "测量值"=w228) -> ("数据标识"=w225:string)  [unwired: 7 in]
            n161 = Bundle By Name(cluster=w230, "数据标识mg/L"=w226, "数据标识%"=w225) -> (w227:T3)
            n162 = global write "多参数全局变量.vi" "DO2显示"(w227) -> ()
          }
          frame "Turb" {
            n163 = global read "断电保存变量.vi" "探头选择"() -> (w262:T7)
            n164 = Unbundle By Name(w262) -> ("浊度探头选择"=w261:T6)
            n165 = global read "多参数全局变量.vi" "MB session in"() -> (w260:refnum<class "MB_Master.lvclass">)
            n166 = case shown="\"STD\"" w261 {
              tunnel: w260 -> [w269 w277 w286 w290]
              tunnel: [w267 w275 w281 w291] -> w254
              tunnel: [w266 w274 w280 w289] -> w259
              frame "禹山", Default {
                n167 = call "禹山浊度_获取温度和测量值.vi"("MB session in"=w269) -> ("error out"=w266:errorcluster, "输出值"=w265:cluster{"温度测量值":sgl, "浊度":sgl})  [unwired: 8 in, 1 out]
                n168 = Unbundle By Name(w265) -> ("温度测量值"=w264:sgl, "浊度"=w263:sgl)
                n169 = global read "多参数全局变量.vi" "浊度显示"() -> (w268:T2)
                n170 = Bundle By Name(cluster=w268, "温度测量值"=w264, "测量值"=w263) -> (w267:T2)
              }
              frame "STD" {
                n171 = call "STD浊度_获取温度和测量值.vi"("MB session in"=w277) -> ("error out"=w274:errorcluster, "STD浊度"=w273:cluster{"温度测量值":sgl, "浊度测量值":sgl, "信号值":sgl})  [unwired: 8 in, 1 out]
                n172 = Unbundle By Name(w273) -> ("温度测量值"=w272:sgl, "浊度测量值"=w271:sgl, "信号值"=w270:sgl)
                n173 = global read "多参数全局变量.vi" "浊度显示"() -> (w276:T2)
                n174 = Bundle By Name(cluster=w276, "温度测量值"=w272, "测量值"=w271, "信号值"=w270) -> (w275:T2)
              }
              frame "国弘" {
                n175 = call "浊度_所有参数读取.vi"("MB session in"=w286) -> ("error out"=w280:errorcluster, "输出值"=w285:T14)  [unwired: 8 in, 1 out]
                n176 = Unbundle By Name(w285) -> ("温度测量值"=w283:sgl, "浊度测量值"=w282:sgl, "温度偏移修正值"=w279:sgl, "浊度信号值"=w278:sgl)
                n177 = global read "多参数全局变量.vi" "浊度显示"() -> (w284:T2)
                n178 = Bundle By Name(cluster=w284, "温度测量值"=w283, "测量值"=w282, "温度偏移修正值"=w279, "信号值"=w278) -> (w281:T2)
              }
              frame "纳清" {
                n179 = call "纳清浊度_所有参数读取.vi"("MB session in"=w290) -> ("error out"=w289:errorcluster, "输出值"=w288:T15)  [unwired: 8 in, 1 out]
                n180 = Unbundle By Name(w288) -> ("温度数据"=w293:sgl, "浊度数值 NTU"=w292:sgl, "原始光强数值"=w287:u16)
                n181 = global read "多参数全局变量.vi" "浊度显示"() -> (w294:T2)
                n182 = Bundle By Name(cluster=w294, "温度测量值"=w293, "测量值"=w292, "信号值"=w287) -> (w291:T2)
              }
            }
            n183 = global read "断电保存变量.vi" "量程参数"() -> (w258:T4)
            n184 = Unbundle By Name(w258) -> ("浊度 (NTU).量程上限"=w257:dbl, "浊度 (NTU).量程下限"=w256:dbl)
            n185 = Unbundle By Name(w254) -> ("测量值"=w253:sgl)
            n186 = Unbundle By Name(w259) -> ("status"=w255:bool)
            n187 = global write "多参数全局变量.vi" "浊度通讯状态"(w255) -> ()
            n188 = call "数据标识判定.vi"("通讯故障"=w255, "量程下限"=w256, "量程上限"=w257, "测量值"=w253) -> ("数据标识"=w251:string)  [unwired: 7 in]
            n189 = Bundle By Name(cluster=w254, "数据标识"=w251) -> (w252:T2)
            n190 = global write "多参数全局变量.vi" "浊度显示"(w252) -> ()
          }
          frame "ORP" {
            n191 = global read "断电保存变量.vi" "探头选择"() -> (w306:T7)
            n192 = Unbundle By Name(w306) -> ("orp探头选择"=w305:T6)
            n193 = global read "多参数全局变量.vi" "MB session in"() -> (w304:refnum<class "MB_Master.lvclass">)
            n194 = case shown="\"禹山\", Default" w305 {
              tunnel: [_ w309 _] -> w303
              tunnel: w304 -> [_ w314 _]
              tunnel: [_ w307 _] -> w298
              frame "禹山", Default {
              }
              frame "国弘" {
                n195 = call "ORP_所有参数读取.vi"("MB session in"=w314) -> ("error out"=w309:errorcluster, "输出值"=w311:T16)  [unwired: 8 in, 1 out]
                n196 = Unbundle By Name(w311) -> ("温度测量值"=w312:sgl, "测量值"=w313:sgl, "信号值"=w308:sgl)
                n197 = global read "多参数全局变量.vi" "ORP显示"() -> (w310:T2)
                n198 = Bundle By Name(cluster=w310, "温度测量值"=w312, "测量值"=w313, "信号值"=w308) -> (w307:T2)
              }
              frame "纳清" {
              }
            }
            n199 = global read "断电保存变量.vi" "量程参数"() -> (w302:T4)
            n200 = Unbundle By Name(w302) -> ("ORP (mV).量程上限"=w301:dbl, "ORP (mV).量程下限"=w300:dbl)
            n201 = Unbundle By Name(w298) -> ("测量值"=w297:sgl)
            n202 = Unbundle By Name(w303) -> ("status"=w299:bool)
            n203 = global write "多参数全局变量.vi" "orp通讯状态"(w299) -> ()
            n204 = call "数据标识判定.vi"("通讯故障"=w299, "量程下限"=w300, "量程上限"=w301, "测量值"=w297) -> ("数据标识"=w295:string)  [unwired: 7 in]
            n205 = Bundle By Name(cluster=w298, "数据标识"=w295) -> (w296:T2)
            n206 = global write "多参数全局变量.vi" "ORP显示"(w296) -> ()
          }
          frame "叶绿素a" {
            n207 = global read "断电保存变量.vi" "探头选择"() -> (w326:T7)
            n208 = Unbundle By Name(w326) -> ("叶绿素a探头选择"=w325:T6)
            n209 = global read "多参数全局变量.vi" "MB session in"() -> (w324:refnum<class "MB_Master.lvclass">)
            n210 = case shown="\"STD\"" w325 {
              tunnel: [w333 w341 _ w347] -> w323
              tunnel: w324 -> [w332 w340 _ w349]
              tunnel: [w330 w338 _ w346] -> w319
              frame "禹山", Default {
                n211 = call "叶绿素a_获取温度和叶绿素值.vi"("MB session in"=w332) -> ("error out"=w333:errorcluster, "输出值"=w329:cluster{"温度测量值":sgl, "叶绿素测量值":sgl, "错误标志":u16})  [unwired: 8 in, 1 out]
                n212 = Unbundle By Name(w329) -> ("温度测量值"=w327:sgl, "叶绿素测量值"=w328:sgl)
                n213 = global read "多参数全局变量.vi" "叶绿素a显示"() -> (w331:T2)
                n214 = Bundle By Name(cluster=w331, "温度测量值"=w327, "测量值"=w328) -> (w330:T2)
              }
              frame "STD" {
                n215 = call "STDchla_获取温度和叶绿素值.vi"("MB session in"=w340) -> ("error out"=w341:errorcluster, "STD叶绿素a"=w337:cluster{"温度测量值":sgl, "叶绿素测量值":sgl, "信号值":sgl})  [unwired: 8 in, 1 out]
                n216 = Unbundle By Name(w337) -> ("温度测量值"=w335:sgl, "叶绿素测量值"=w336:sgl, "信号值"=w334:sgl)
                n217 = global read "多参数全局变量.vi" "叶绿素a显示"() -> (w339:T2)
                n218 = Bundle By Name(cluster=w339, "温度测量值"=w335, "测量值"=w336, "信号值"=w334) -> (w338:T2)
              }
              frame "国弘" {
              }
              frame "纳清" {
                n219 = call "纳清叶绿素a_所有参数读取.vi"("MB session in"=w349) -> ("error out"=w347:errorcluster, "输出值"=w345:T17)  [unwired: 8 in, 1 out]
                n220 = Unbundle By Name(w345) -> ("温度数据"=w343:sgl, "叶绿素a"=w344:sgl, "原始光强数值"=w342:u16)
                n221 = global read "多参数全局变量.vi" "叶绿素a显示"() -> (w348:T2)
                n222 = Bundle By Name(cluster=w348, "温度测量值"=w343, "测量值"=w344, "信号值"=w342) -> (w346:T2)
              }
            }
            n223 = global read "断电保存变量.vi" "量程参数"() -> (w322:T4)
            n224 = Unbundle By Name(w322) -> ("叶绿素a (μg/L).量程上限"=w321:dbl, "叶绿素a (μg/L).量程下限"=w320:dbl)
            n225 = Unbundle By Name(w319) -> ("测量值"=w318:sgl)
            n226 = Unbundle By Name(w323) -> ("status"=w317:bool)
            n227 = global write "多参数全局变量.vi" "叶绿素a通讯状态"(w317) -> ()
            n228 = call "数据标识判定.vi"("通讯故障"=w317, "量程下限"=w320, "量程上限"=w321, "测量值"=w318) -> ("数据标识"=w315:string)  [unwired: 7 in]
            n229 = Bundle By Name(cluster=w319, "数据标识"=w315) -> (w316:T2)
            n230 = global write "多参数全局变量.vi" "叶绿素a显示"(w316) -> ()
          }
          frame "藻密度" {
            n231 = global read "断电保存变量.vi" "探头选择"() -> (w361:T7)
            n232 = Unbundle By Name(w361) -> ("蓝绿藻探头选择"=w360:T6)
            n233 = global read "多参数全局变量.vi" "MB session in"() -> (w359:refnum<class "MB_Master.lvclass">)
            n234 = case shown="\"STD\"" w360 {
              tunnel: [_ w363 _ w375] -> w358
              tunnel: w359 -> [_ w364 _ w377]
              tunnel: [_ w362 _ w374] -> w354
              frame "禹山", Default {
              }
              frame "STD" {
                n235 = call "STDBGA_获取温度和叶绿素值.vi"("MB session in"=w364) -> ("error out"=w363:errorcluster, "STD藻密度"=w368:cluster{"温度测量值":sgl, "测试值":dbl, "信号值":sgl})  [unwired: 8 in, 1 out]
                n236 = Unbundle By Name(w368) -> ("温度测量值"=w366:sgl, "测试值"=w367:dbl, "信号值"=w365:sgl)
                n237 = global read "多参数全局变量.vi" "藻密度显示"() -> (w369:T2)
                n238 = Bundle By Name(cluster=w369, "温度测量值"=w366, "测量值"=w367, "信号值"=w365) -> (w362:T2)
              }
              frame "国弘" {
              }
              frame "纳清" {
                n239 = call "纳清蓝绿藻_所有参数读取.vi"("MB session in"=w377) -> ("error out"=w375:errorcluster, "输出值"=w373:T18)  [unwired: 8 in, 1 out]
                n240 = Unbundle By Name(w373) -> ("温度数据"=w372:sgl, "蓝绿藻"=w371:sgl, "原始光强数值"=w370:u16)
                n241 = global read "多参数全局变量.vi" "藻密度显示"() -> (w376:T2)
                n242 = Bundle By Name(cluster=w376, "温度测量值"=w372, "测量值"=w371, "信号值"=w370) -> (w374:T2)
              }
            }
            n243 = global read "断电保存变量.vi" "量程参数"() -> (w357:T4)
            n244 = Unbundle By Name(w357) -> ("藻密度 (cells/mL).量程上限"=w356:dbl, "藻密度 (cells/mL).量程下限"=w355:dbl)
            n245 = Unbundle By Name(w354) -> ("测量值"=w353:sgl)
            n246 = Unbundle By Name(w358) -> ("status"=w352:bool)
            n247 = global write "多参数全局变量.vi" "藻密度通讯状态"(w352) -> ()
            n248 = call "数据标识判定.vi"("通讯故障"=w352, "量程下限"=w355, "量程上限"=w356, "测量值"=w353) -> ("数据标识"=w350:string)  [unwired: 7 in]
            n249 = Bundle By Name(cluster=w354, "数据标识"=w350) -> (w351:T2)
            n250 = global write "多参数全局变量.vi" "藻密度显示"(w351) -> ()
          }
          frame "COD" {
            n251 = global read "断电保存变量.vi" "探头选择"() -> (w389:T7)
            n252 = Unbundle By Name(w389) -> ("COD探头选择"=w388:T6)
            n253 = global read "多参数全局变量.vi" "MB session in"() -> (w387:refnum<class "MB_Master.lvclass">)
            n254 = case shown="\"禹山\", Default" w388 {
              tunnel: [_ w395 _] -> w386
              tunnel: w387 -> [_ w397 _]
              tunnel: [_ w394 _] -> w385
              frame "禹山", Default {
              }
              frame "国弘" {
                n255 = call "COD_所有参数读取.vi"("MB session in"=w397) -> ("error out"=w395:errorcluster, "输出值"=w393:T19)  [unwired: 8 in, 1 out]
                n256 = Unbundle By Name(w393) -> ("温度测量值"=w392:sgl, "COD测量值"=w391:sgl, "COD信号值"=w390:sgl)
                n257 = global read "多参数全局变量.vi" "COD显示"() -> (w396:T2)
                n258 = Bundle By Name(cluster=w396, "温度测量值"=w392, "测量值"=w391, "信号值"=w390) -> (w394:T2)
              }
              frame "纳清" {
              }
            }
            n259 = global read "断电保存变量.vi" "量程参数"() -> (w380:T4)
            n260 = Unbundle By Name(w385) -> ("测量值"=w384:sgl)
            n261 = Unbundle By Name(w380) -> ("COD.量程上限"=w379:dbl, "COD.量程下限"=w378:dbl)
            n262 = Unbundle By Name(w386) -> ("status"=w383:bool)
            n263 = global write "多参数全局变量.vi" "cod通讯状态"(w383) -> ()
            n264 = call "数据标识判定.vi"("通讯故障"=w383, "量程下限"=w378, "量程上限"=w379, "测量值"=w384) -> ("数据标识"=w381:string)  [unwired: 7 in]
            n265 = Bundle By Name(cluster=w385, "数据标识"=w381) -> (w382:T2)
            n266 = global write "多参数全局变量.vi" "COD显示"(w382) -> ()
          }
          frame "氯化物" {
            n267 = global read "多参数全局变量.vi" "MB session in"() -> (w412:refnum<class "MB_Master.lvclass">)
            n268 = call "氯化物_所有参数读取.vi"("MB session in"=w412) -> ("error out"=w411:errorcluster, "输出值"=w404:T20)  [unwired: 8 in, 1 out]
            n269 = Unbundle By Name(w404) -> ("温度测量值"=w403:sgl, "测量值"=w402:sgl, "信号值"=w401:sgl)
            n270 = global read "多参数全局变量.vi" "氯化物显示"() -> (w405:T2)
            n271 = Unbundle By Name(w411) -> ("status"=w408:bool)
            n272 = global write "多参数全局变量.vi" "氯化物通讯状态"(w408) -> ()
            n273 = Bundle By Name(cluster=w405, "温度测量值"=w403, "测量值"=w402, "信号值"=w401) -> (w410:T2)
            n274 = global read "断电保存变量.vi" "量程参数"() -> (w400:T4)
            n275 = Unbundle By Name(w400) -> ("氯化物（mg/L）.量程上限"=w399:dbl, "氯化物（mg/L）.量程下限"=w398:dbl)
            n276 = Unbundle By Name(w410) -> ("测量值"=w409:sgl)
            n277 = call "数据标识判定.vi"("通讯故障"=w408, "量程下限"=w398, "量程上限"=w399, "测量值"=w409) -> ("数据标识"=w406:string)  [unwired: 7 in]
            n278 = Bundle By Name(cluster=w410, "数据标识"=w406) -> (w407:T2)
            n279 = global write "多参数全局变量.vi" "氯化物显示"(w407) -> ()
          }
          frame "水中油" {
            n280 = global read "多参数全局变量.vi" "MB session in"() -> (w415:refnum<class "MB_Master.lvclass">)
            n281 = call "水中油_所有参数读取.vi"("MB session in"=w415) -> ("error out"=w413:errorcluster, "输出值"=w414:T21)  [unwired: 8 in, 1 out]
            n282 = Unbundle By Name(w414) -> ("温度测量值"=w421:sgl, "测量值"=w420:sgl, "信号值"=w419:sgl)
            n283 = global read "多参数全局变量.vi" "水中油显示"() -> (w422:T2)
            n284 = Unbundle By Name(w413) -> ("status"=w425:bool)
            n285 = global write "多参数全局变量.vi" "水中油通讯状态"(w425) -> ()
            n286 = Bundle By Name(cluster=w422, "温度测量值"=w421, "测量值"=w420, "信号值"=w419) -> (w427:T2)
            n287 = global read "断电保存变量.vi" "量程参数"() -> (w418:T4)
            n288 = Unbundle By Name(w418) -> ("水中油.量程上限"=w417:dbl, "水中油.量程下限"=w416:dbl)
            n289 = Unbundle By Name(w427) -> ("测量值"=w426:sgl)
            n290 = call "数据标识判定.vi"("通讯故障"=w425, "量程下限"=w416, "量程上限"=w417, "测量值"=w426) -> ("数据标识"=w423:string)  [unwired: 7 in]
            n291 = Bundle By Name(cluster=w427, "数据标识"=w423) -> (w424:T2)
            n292 = global write "多参数全局变量.vi" "水中油显示"(w424) -> ()
          }
          frame "氨氮" {
            n293 = global read "多参数全局变量.vi" "MB session in"() -> (w430:refnum<class "MB_Master.lvclass">)
            n294 = call "纳清氨氮_所有参数读取.vi"("MB session in"=w430) -> ("error out"=w428:errorcluster, "输出值"=w429:T22)  [unwired: 8 in, 1 out]
            n295 = Unbundle By Name(w429) -> ("温度数据"=w436:sgl, "参数2数据"=w435:sgl, "参数2原始信号"=w434:sgl)
            n296 = Unbundle By Name(w428) -> ("status"=w440:bool)
            n297 = global read "多参数全局变量.vi" "氨氮显示"() -> (w437:T2)
            n298 = global write "多参数全局变量.vi" "氨氮通讯状态"(w440) -> ()
            n299 = Bundle By Name(cluster=w437, "温度测量值"=w436, "测量值"=w435, "信号值"=w434) -> (w442:T2)
            n300 = global read "断电保存变量.vi" "量程参数"() -> (w433:T4)
            n301 = Unbundle By Name(w442) -> ("测量值"=w441:sgl)
            n302 = Unbundle By Name(w433) -> ("氨氮.量程上限"=w432:dbl, "氨氮.量程下限"=w431:dbl)
            n303 = call "数据标识判定.vi"("通讯故障"=w440, "量程下限"=w431, "量程上限"=w432, "测量值"=w441) -> ("数据标识"=w438:string)  [unwired: 7 in]
            n304 = Bundle By Name(cluster=w442, "数据标识"=w438) -> (w439:T2)
            n305 = global write "多参数全局变量.vi" "氨氮显示"(w439) -> ()
          }
        }
      }
      frame #2 {
        n306 = Format Date/Time String() -> (date/time string=→"日期/时间字符串 2":string)  [unwired: 3 in]
        n307 = Wait (ms)(milliseconds to wait=u32 500 ("等待时间（毫秒）")) -> ()  [unwired: 1 out]
      }
    }
  }
  n308 = while {
    tunnel: w1 -> [w626]
    stop <- FALSE stop-if-true
    w526 = T1[] [enum."pH", enum."DO", enum."Cond", enum."Turb", enum."ORP", enum."叶绿素a", enum."藻密度", enum."COD", enum."DO2", enum."氯化物", enum."氨氮", enum."水中油"] items=["pH", "DO", "DO2", "Cond", "Turb", "ORP", "叶绿素a", "藻密度", "COD", "氯化物", "氨氮", "水中油"]
    n309 = global read "多参数全局变量.vi" "远程校准运行状态"() -> (w623:T23)
    n310 = global read "多参数全局变量.vi" "远程校准运行状态"() -> (w597:T23)
    n311 = global read "多参数全局变量.vi" "远程校准运行状态"() -> (w600:T23)
    n312 = global read "多参数全局变量.vi" "远程校准运行状态"() -> (w584:T23)
    n313 = global read "多参数全局变量.vi" "远程校准运行状态"() -> (w571:T23)
    n314 = global read "多参数全局变量.vi" "远程校准运行状态"() -> (w514:T23)
    n315 = global read "多参数全局变量.vi" "远程校准运行状态"() -> (w496:T23)
    n316 = global read "多参数全局变量.vi" "远程校准运行状态"() -> (w460:T23)
    n317 = global read "多参数全局变量.vi" "校准运行状态"() -> (w612:T24)
    n318 = global read "多参数全局变量.vi" "校准运行状态"() -> (w586:T24)
    n319 = global read "多参数全局变量.vi" "校准运行状态"() -> (w611:T24)
    n320 = global read "多参数全局变量.vi" "校准运行状态"() -> (w573:T24)
    n321 = global read "多参数全局变量.vi" "校准运行状态"() -> (w560:T24)
    n322 = global read "多参数全局变量.vi" "校准运行状态"() -> (w521:T24)
    n323 = global read "多参数全局变量.vi" "校准运行状态"() -> (w507:T24)
    n324 = global read "多参数全局变量.vi" "校准运行状态"() -> (w471:T24)
    n325 = global read "多参数全局变量.vi" "远程校准运行状态"() -> (w548:T23)
    n326 = global read "多参数全局变量.vi" "远程校准运行状态"() -> (w545:T23)
    n327 = global read "多参数全局变量.vi" "远程校准运行状态"() -> (w486:T23)
    n328 = global read "多参数全局变量.vi" "远程校准运行状态"() -> (w458:T23)
    n329 = global read "多参数全局变量.vi" "校准运行状态"() -> (w559:T24)
    n330 = global read "多参数全局变量.vi" "校准运行状态"() -> (w534:T24)
    n331 = global read "多参数全局变量.vi" "校准运行状态"() -> (w475:T24)
    n332 = global read "多参数全局变量.vi" "校准运行状态"() -> (w447:T24)
    n333 = Unbundle By Name(w611) -> ("Cond"=w609:bool)
    n334 = Unbundle By Name(w600) -> ("Cond"=w601:bool)
    n335 = Unbundle By Name(w573) -> ("Turb"=w575:bool)
    n336 = Unbundle By Name(w584) -> ("Turb"=w583:bool)
    n337 = Unbundle By Name(w521) -> ("COD"=w520:bool)
    n338 = Unbundle By Name(w507) -> ("DO2"=w505:bool)
    n339 = Unbundle By Name(w496) -> ("DO2"=w497:bool)
    n340 = Unbundle By Name(w560) -> ("ORP"=w562:bool)
    n341 = Unbundle By Name(w571) -> ("ORP"=w570:bool)
    n342 = Unbundle By Name(w514) -> ("cod"=w515:bool)
    n343 = Unbundle By Name(w471) -> ("氨氮"=w469:bool)
    n344 = Unbundle By Name(w460) -> ("氨氮"=w462:bool)
    n345 = Unbundle By Name(w586) -> ("DO"=w588:bool)
    n346 = Unbundle By Name(w597) -> ("DO"=w596:bool)
    n347 = Unbundle By Name(w612) -> ("ph"=w614:bool)
    n348 = Unbundle By Name(w623) -> ("ph"=w622:bool)
    n349 = Cluster To Array(cluster=w612) -> (array=w617:bool[])
    n350 = Cluster To Array(cluster=w623) -> (array=w619:bool[])
    n351 = Cluster To Array(cluster=w586) -> (array=w591:bool[])
    n352 = Cluster To Array(cluster=w597) -> (array=w593:bool[])
    n353 = Cluster To Array(cluster=w611) -> (array=w606:bool[])
    n354 = Cluster To Array(cluster=w600) -> (array=w604:bool[])
    n355 = Cluster To Array(cluster=w573) -> (array=w578:bool[])
    n356 = Cluster To Array(cluster=w584) -> (array=w580:bool[])
    n357 = Cluster To Array(cluster=w560) -> (array=w565:bool[])
    n358 = Cluster To Array(cluster=w571) -> (array=w567:bool[])
    n359 = Cluster To Array(cluster=w521) -> (array=w517:bool[])
    n360 = Cluster To Array(cluster=w514) -> (array=w513:bool[])
    n361 = Cluster To Array(cluster=w507) -> (array=w502:bool[])
    n362 = Cluster To Array(cluster=w496) -> (array=w500:bool[])
    n363 = Cluster To Array(cluster=w471) -> (array=w470:bool[])
    n364 = Cluster To Array(cluster=w460) -> (array=w461:bool[])
    n365 = Unbundle By Name(w559) -> ("叶绿素a"=w557:bool)
    n366 = Unbundle By Name(w548) -> ("叶绿素a"=w549:bool)
    n367 = Unbundle By Name(w534) -> ("藻密度"=w536:bool)
    n368 = Unbundle By Name(w545) -> ("藻密度"=w544:bool)
    n369 = Unbundle By Name(w475) -> ("氯化物"=w477:bool)
    n370 = Unbundle By Name(w486) -> ("氯化物"=w484:bool)
    n371 = Unbundle By Name(w447) -> ("水中油"=w449:bool)
    n372 = Unbundle By Name(w458) -> ("水中油"=w456:bool)
    n373 = Boolean Array To Number(Boolean array=w617) -> (number=w616:u32)
    n374 = Boolean Array To Number(Boolean array=w619) -> (number=w620:u32)
    n375 = Boolean Array To Number(Boolean array=w591) -> (number=w590:u32)
    n376 = Boolean Array To Number(Boolean array=w593) -> (number=w594:u32)
    n377 = Boolean Array To Number(Boolean array=w606) -> (number=w607:u32)
    n378 = Boolean Array To Number(Boolean array=w604) -> (number=w603:u32)
    n379 = Boolean Array To Number(Boolean array=w578) -> (number=w577:u32)
    n380 = Boolean Array To Number(Boolean array=w580) -> (number=w581:u32)
    n381 = Boolean Array To Number(Boolean array=w565) -> (number=w564:u32)
    n382 = Boolean Array To Number(Boolean array=w567) -> (number=w568:u32)
    n383 = Boolean Array To Number(Boolean array=w517) -> (number=w518:u32)
    n384 = Boolean Array To Number(Boolean array=w513) -> (number=w512:u32)
    n385 = Boolean Array To Number(Boolean array=w502) -> (number=w503:u32)
    n386 = Boolean Array To Number(Boolean array=w500) -> (number=w499:u32)
    n387 = Boolean Array To Number(Boolean array=w470) -> (number=w468:u32)
    n388 = Boolean Array To Number(Boolean array=w461) -> (number=w463:u32)
    n389 = Cluster To Array(cluster=w559) -> (array=w554:bool[])
    n390 = Cluster To Array(cluster=w548) -> (array=w552:bool[])
    n391 = Cluster To Array(cluster=w534) -> (array=w539:bool[])
    n392 = Cluster To Array(cluster=w545) -> (array=w541:bool[])
    n393 = Cluster To Array(cluster=w475) -> (array=w476:bool[])
    n394 = Cluster To Array(cluster=w486) -> (array=w485:bool[])
    n395 = Cluster To Array(cluster=w447) -> (array=w448:bool[])
    n396 = Cluster To Array(cluster=w458) -> (array=w457:bool[])
    n397 = Equal To 0?(x=w616) -> (x = 0?=w615:bool)
    n398 = Equal To 0?(x=w620) -> (x = 0?=w621:bool)
    n399 = Equal To 0?(x=w590) -> (x = 0?=w589:bool)
    n400 = Equal To 0?(x=w594) -> (x = 0?=w595:bool)
    n401 = Equal To 0?(x=w607) -> (x = 0?=w608:bool)
    n402 = Equal To 0?(x=w603) -> (x = 0?=w602:bool)
    n403 = Equal To 0?(x=w577) -> (x = 0?=w576:bool)
    n404 = Equal To 0?(x=w581) -> (x = 0?=w582:bool)
    n405 = Equal To 0?(x=w564) -> (x = 0?=w563:bool)
    n406 = Equal To 0?(x=w568) -> (x = 0?=w569:bool)
    n407 = Equal To 0?(x=w518) -> (x = 0?=w519:bool)
    n408 = Equal To 0?(x=w512) -> (x = 0?=w516:bool)
    n409 = Equal To 0?(x=w503) -> (x = 0?=w504:bool)
    n410 = Equal To 0?(x=w499) -> (x = 0?=w498:bool)
    n411 = Equal To 0?(x=w468) -> (x = 0?=w467:bool)
    n412 = Equal To 0?(x=w463) -> (x = 0?=w464:bool)
    n413 = Boolean Array To Number(Boolean array=w554) -> (number=w555:u32)
    n414 = Boolean Array To Number(Boolean array=w552) -> (number=w551:u32)
    n415 = Boolean Array To Number(Boolean array=w539) -> (number=w538:u32)
    n416 = Boolean Array To Number(Boolean array=w541) -> (number=w542:u32)
    n417 = Boolean Array To Number(Boolean array=w476) -> (number=w478:u32)
    n418 = Boolean Array To Number(Boolean array=w485) -> (number=w483:u32)
    n419 = Boolean Array To Number(Boolean array=w448) -> (number=w450:u32)
    n420 = Boolean Array To Number(Boolean array=w457) -> (number=w455:u32)
    n421 = Or(x=w614, y=w615) -> (x .or. y?=w613:bool)
    n422 = Or(x=w622, y=w621) -> (x .or. y?=w624:bool)
    n423 = Or(x=w588, y=w589) -> (x .or. y?=w587:bool)
    n424 = Or(x=w596, y=w595) -> (x .or. y?=w598:bool)
    n425 = Or(x=w609, y=w608) -> (x .or. y?=w610:bool)
    n426 = Or(x=w601, y=w602) -> (x .or. y?=w599:bool)
    n427 = Or(x=w575, y=w576) -> (x .or. y?=w574:bool)
    n428 = Or(x=w583, y=w582) -> (x .or. y?=w585:bool)
    n429 = Or(x=w562, y=w563) -> (x .or. y?=w561:bool)
    n430 = Or(x=w570, y=w569) -> (x .or. y?=w572:bool)
    n431 = Or(x=w520, y=w519) -> (x .or. y?=w511:bool)
    n432 = Or(x=w515, y=w516) -> (x .or. y?=w510:bool)
    n433 = Or(x=w505, y=w504) -> (x .or. y?=w506:bool)
    n434 = Or(x=w497, y=w498) -> (x .or. y?=w495:bool)
    n435 = Or(x=w469, y=w467) -> (x .or. y?=w472:bool)
    n436 = Or(x=w462, y=w464) -> (x .or. y?=w466:bool)
    n437 = Equal To 0?(x=w555) -> (x = 0?=w556:bool)
    n438 = Equal To 0?(x=w551) -> (x = 0?=w550:bool)
    n439 = Equal To 0?(x=w538) -> (x = 0?=w537:bool)
    n440 = Equal To 0?(x=w542) -> (x = 0?=w543:bool)
    n441 = Equal To 0?(x=w478) -> (x = 0?=w479:bool)
    n442 = Equal To 0?(x=w483) -> (x = 0?=w482:bool)
    n443 = Equal To 0?(x=w450) -> (x = 0?=w451:bool)
    n444 = Equal To 0?(x=w455) -> (x = 0?=w454:bool)
    n445 = global read "断电保存变量.vi" "叶绿素a启用"() -> (w553:bool)
    n446 = global read "断电保存变量.vi" "藻密度"() -> (w540:bool)
    n447 = global read "断电保存变量.vi" "氯化物"() -> (w481:bool)
    n448 = global read "断电保存变量.vi" "水中油"() -> (w453:bool)
    n449 = global read "断电保存变量.vi" "Cond"() -> (w605:bool)
    n450 = global read "断电保存变量.vi" "DO 2"() -> (w501:bool)
    n451 = global read "断电保存变量.vi" "Turb"() -> (w579:bool)
    n452 = global read "断电保存变量.vi" "COD"() -> (w522:bool)
    n453 = Or(x=w557, y=w556) -> (x .or. y?=w558:bool)
    n454 = Or(x=w549, y=w550) -> (x .or. y?=w547:bool)
    n455 = Or(x=w536, y=w537) -> (x .or. y?=w535:bool)
    n456 = Or(x=w544, y=w543) -> (x .or. y?=w546:bool)
    n457 = Or(x=w477, y=w479) -> (x .or. y?=w474:bool)
    n458 = Or(x=w484, y=w482) -> (x .or. y?=w480:bool)
    n459 = global read "断电保存变量.vi" "氨氮"() -> (w465:bool)
    n460 = Or(x=w449, y=w451) -> (x .or. y?=w446:bool)
    n461 = Or(x=w456, y=w454) -> (x .or. y?=w452:bool)
    n462 = global read "断电保存变量.vi" "orp"() -> (w566:bool)
    n463 = global read "断电保存变量.vi" "DO"() -> (w592:bool)
    n464 = global read "断电保存变量.vi" "pH"() -> (w618:bool)
    n465 = Compound Arithmetic op=AND ("复合运算")(w618, w613, w624) -> (w533:bool)
    n466 = Compound Arithmetic op=AND ("复合运算")(w592, w587, w598) -> (w508:bool)
    n467 = Compound Arithmetic op=AND ("复合运算")(w605, w610, w599) -> (w532:bool)
    n468 = Compound Arithmetic op=AND ("复合运算")(w579, w574, w585) -> (w531:bool)
    n469 = Compound Arithmetic op=AND ("复合运算")(w566, w561, w572) -> (w530:bool)
    n470 = Compound Arithmetic op=AND ("复合运算")(w553, w558, w547) -> (w529:bool)
    n471 = Compound Arithmetic op=AND ("复合运算")(w540, w535, w546) -> (w528:bool)
    n472 = Compound Arithmetic op=AND ("复合运算")(w522, w511, w510) -> (w509:bool)
    n473 = Compound Arithmetic op=AND ("复合运算")(w501, w506, w495) -> (w494:bool)
    n474 = Compound Arithmetic op=AND ("复合运算")(w481, w474, w480) -> (w473:bool)
    n475 = Compound Arithmetic op=AND ("复合运算")(w465, w472, w466) -> (w459:bool)
    n476 = Compound Arithmetic op=AND ("复合运算")(w453, w446, w452) -> (w445:bool)
    n477 = Build Array(w533, w508, w532, w531, w530, w529, w528, w509, w494, w473, w459, w445) -> (w527:bool[])
    n478 = for {
      tunnel: w527 -> [w632] mode=indexing
      tunnel: w526 -> [w633] mode=indexing
      tunnel: [w633] -> w525 mode=indexing if=w632
      tunnel: [w631] -> w493
      i -> [w631]
    }
    n479 = Less Or Equal?(x=w493, y=1) -> (x <= y?=w491:bool)
    n480 = Select(t=u32 2000 ("等待时间（毫秒）"), s=w491, f=u32 1000 ("等待时间（毫秒）")) -> (s? t:f=w488:u32)
    n481 = Wait (ms)(milliseconds to wait=w488) -> (millisecond timer value=w487:u32)
    n482 = Get Queue Status(queue=w626) -> (queue out=w524:refnum<queue>, # elements in queue=w523:i32)  [unwired: 2 in, 6 out]
    n483 = case shown="0" w523 {
      tunnel: w525 -> [_ w628]
      tunnel: w524 -> [_ w627]
      tunnel: w487 -> [_ _]
      frame Default {
      }
      frame 0 {
        n484 = for {
          tunnel: w627 -> [w630]
          tunnel: w628 -> [w629] mode=indexing
          n485 = Enqueue Element(queue=w630, element=w629) -> ()  [unwired: 2 in, 3 out]
        }
      }
    }
  }
